vi "test 2.vi"() -> ()   [LabVIEW 2012, in "Data Logger.lvlib"]
uses:
  Data Logger.lvlib
panel:
  out "i3":i32
  out "i2":i32
  out "i1":i32
  in  "stop":bool
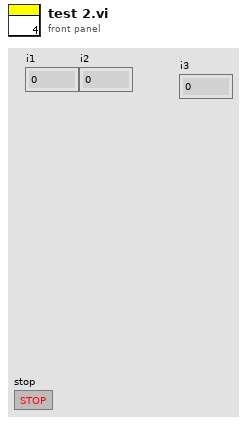
[diagram p1: front panel]
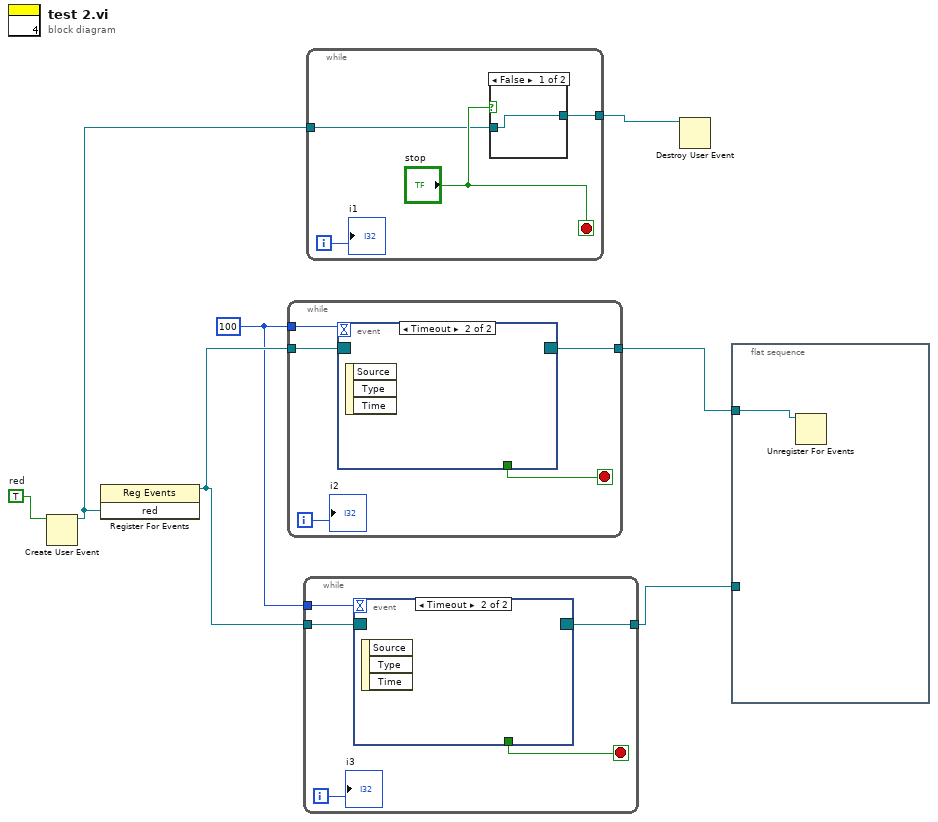
[diagram p0: block diagram]
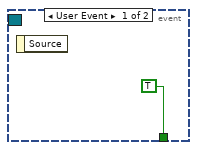
[diagram p2: hidden frame]
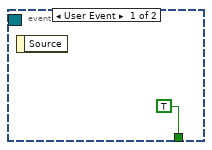
[diagram p3: hidden frame]
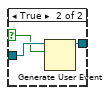
[diagram p4: hidden frame]
diagram:
  w1 = 100
  w7 = TRUE  # red
  n1 = Create User Event(user event datatype=w7) -> (user event=w6:refnum<user-event>)  [unwired: 1 in, 1 out]
  n2 = register-events(w6) -> (reference out=w4:refnum<event-registration>)  [unwired: 2 in, 1 out]
  n3 = while {
    tunnel: w4 -> [w12]
    tunnel: [w11] -> w3
    tunnel: w1 -> [w8]
    i -> [w9]
    stop <- w10 stop-if-true
    n4 = event shown="[1] Timeout" {
      selector: w12 -> [_ _]
      dyn-events: [_ _] -> w11
      timeout: w8 -> [_ _]
      tunnel: [TRUE _] -> w10
      event User Event {
        n5 = event-data() -> ()  [unwired: 1 in, 1 out]
      }
      event Timeout {
        n6 = event-data() -> ()  [unwired: 1 in, 3 out]
      }
    }
    "i2" <- w9
  }
  n7 = while {
    tunnel: w4 -> [w18]
    tunnel: [w17] -> w2
    tunnel: w1 -> [w14]
    i -> [w15]
    stop <- w16 stop-if-true
    n8 = event shown="[1] Timeout" {
      selector: w18 -> [_ _]
      dyn-events: [_ _] -> w17
      timeout: w14 -> [_ _]
      tunnel: [TRUE _] -> w16
      event User Event {
        n9 = event-data() -> ()  [unwired: 1 in, 1 out]
      }
      event Timeout {
        n10 = event-data() -> ()  [unwired: 1 in, 3 out]
      }
    }
    "i3" <- w15
  }
  n11 = while {
    tunnel: w6 -> [w22]
    tunnel: [w21] -> w5
    i -> [w20]
    stop <- "stop" stop-if-true
    n12 = case shown="False" "stop" {
      selector: "stop" -> [_ w26]
      tunnel: w22 -> [w24 w27]
      tunnel: [w24 w25] -> w21
      frame False {
      }
      frame True {
        n13 = Generate User Event(user event=w27, event data cluster=w26) -> (user event out=w25:refnum<user-event>)  [unwired: 1 in, 1 out]
      }
    }
    "i1" <- w20
  }
  n14 = Destroy User Event(user event=w5) -> ()  [unwired: 1 in, 1 out]
  n15 = flat-sequence {
    tunnel: w3 -> [w28]
    tunnel: w2 -> [_]
    frame #0 {
      n16 = Unregister For Events(event registration refnum=w28) -> ()  [unwired: 1 in, 1 out]
    }
  }
